vi "zlgcan_demo_USBCANFD_merge.vi"() -> ()   [LabVIEW 2018]
doc: "用于设置CAN通道的初始化参数。\n\n适用的设备：USBCANFD-100U、USBCANFD-200U、USBCANFD-MINI"
uses:
  data_type/ZCAN_InitCAN_setting_USBCANFD.ctl
  data_type/ZCAN_TransmitFD_frame.ctl
  data_type/ZCANDataObj.ctl
panel:
  out "CAN报文显示":string[][](table)
  in  "ZCANDataObj":T1[](array[typedef])
  in  "canfdframe":T2
  out "source":string
  in  "开启CAN":bool
  in  "stop":bool
  in  "?":enum32{"DEMO说明", "设备、通道选择", "参数设置", "状态", "发送"}(tab)
  in  "CAN 通道":u32(ring) items=["0", "1"]
  in  "CAN卡型号":u32(ring)=42 items=["USBCANFD-800U"=59, "USBCANFD-200U"=41, "USBCANFD-100U"=42, "USBCANFD-MINI"=43]
  in  "索引":u32(ring) items=["0", "1", "2", "3", "4", "5", "6", "7", "8"]
  in  "仲裁域波特率":u32(ring)=500000 items=["1Mbps"=1000000, "800kbps"=800000, "500kbps"=500000, "250kbps"=250000, "125kbps"=125000, "100kbps"=100000, "50kbps"=50000]
  in  "数据域波特率":u32(ring)=500000 items=["5Mbps"=5000000, "4Mbps"=4000000, "2Mbps"=2000000, "1Mbps"=1000000, "800kbps"=800000, "500kbps"=500000, "250kbps"=250000, "125kbps"=125000, "100kbps"=100000]
  in  "自定义波特率字符输入":string
  in  "自定义波特率开关":bool
  in  "工作模式":u8(ring) items=["正常", "只听"]
  in  "是否使用电阻":u8(ring)=1 items=["不使用终端电阻", "使用终端电阻"]
  out "error out":errorcluster caption="错误输出"
  out "can_index_handle(out)":u32
  out "Device_handle(out)":u32
  in  "帧类型":u32(ring) items=["标准帧", "扩展帧"]
  in  "帧格式":u32(ring) items=["数据帧", "远程帧"]
  in  "ID":u32=18 format="0x%08x"
  in  "协议":u32(ring) items=["CAN", "CANFD"]
  in  "数据输入":string="11 22 33 44 55 66 77 88"
  in  "CANFD加速？":u32(ring) items=["不加速", "加速"]
  in  "发送":bool
  in  "数据长度":u32(ring)=8 items=["1"=1, "2"=2, "3"=3, "4"=4, "5"=5, "6"=6, "7"=7, "8"=8, "12"=12, "16"=16, "20"=20, "24"=24, "32"=32, "48"=48, "64"=64]
  in  "ZCAN_InitCAN_Setting_USBCANFD":T3
  # "适用的设备：USBCANFD-100U、USBCANFD-200U、USBCANFD-MINI、USBCANFD-800U"
  # "停止程序前，\n请先关闭CAN卡"
  # "1. 确保电脑有VC++ 2005/2008/2010/2013运行库（对应32，64位）,微软常用运行库合集，点击下载（35M）。\n    http://manual.zlg.cn/Public/Uploads/2020-06-05/5ed995c271414.zip"
  # "2，如果打开设备失败，可能原因：\n（1）已经打开过一次，没有正常关闭的情况下，继续点击“打开设备”，是无法打开的。\n     需要USB重新拔插，LABVIEW重启（全部关闭），然后再“打开设备”。\n (2) 项目路径不能有中文繁体。"
  # "使用CAN时，\n两个波特率设置相同即可"
  # "使用ZCANPro软件波特率计算工具计算"
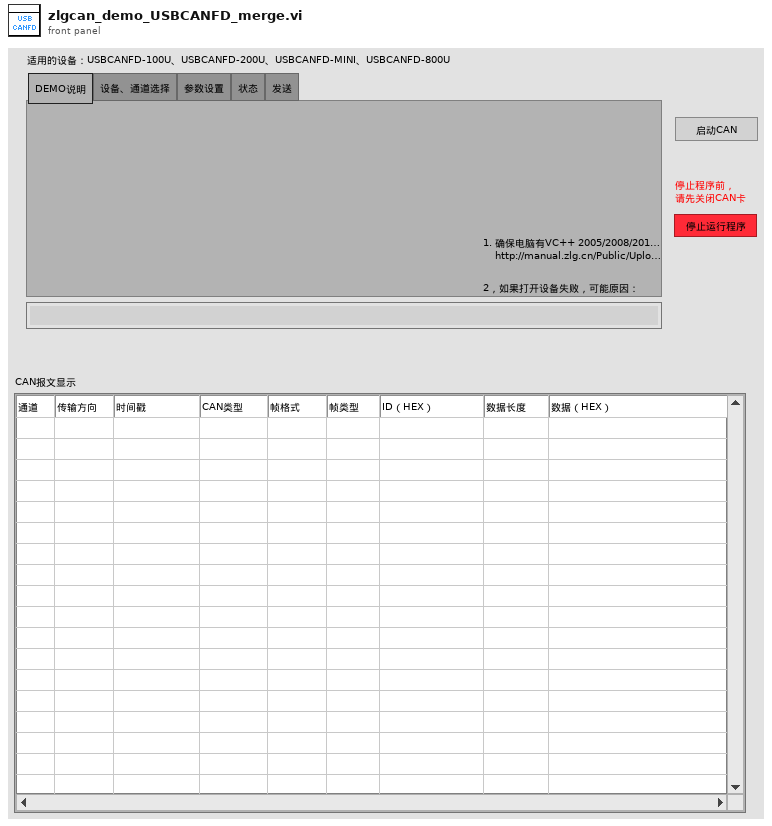
[diagram p1: front panel]
types:
  T1 = typedef "ZCANDataObj.ctl" = cluster{"数据类型":u8, "CAN通道号":u8, "rawVal(未使用)":u16, "extraData[4]（未使用）":cluster{"[0]":u8, "[1]":u8, "[2]":u8, "[3]":u8}, "canCANFDData":cluster{"时间戳+混合标志位":cluster{"时间戳":u64, "混合标志位":u32}, "extraData[4]（未使用）":cluster{"[0]":u8, "[1]":u8, "[2]":u8, "[3]":u8}, "frame":cluster{"can_id":u32, "数据长度":u8, "CANFD加速？":u8, "__res0":u8, "__res1":u8, "data":cluster{"CAN数据[0]":u8, "CAN数据[1]":u8, "CAN数据[2]":u8, "CAN数据[3]":u8, "CAN数据[4]":u8, "CAN数据[5]":u8, "CAN数据[6]":u8, "CAN数据[7]":u8, "CAN数据[8]":u8, "CAN数据[9]":u8, "CAN数据[10]":u8, "CAN数据[11] ":u8, "CAN数据[12] ":u8, "CAN数据[13] ":u8, "CAN数据[14] ":u8, "CAN数据[15] ":u8, "CAN数据[16]":u8, "CAN数据[17]":u8, "CAN数据[18]":u8, "CAN数据[19]":u8, "CAN数据[20]":u8, "CAN数据[21]":u8, "CAN数据[22]":u8, "CAN数据[23]":u8, "CAN数据[24] ":u8, "CAN数据[25]":u8, "CAN数据[26]":u8, "CAN数据[27]":u8, "CAN数据[28]":u8, "CAN数据[29]":u8, "CAN数据[30]":u8, "CAN数据[31]":u8, "CAN数据[32]":u8, "CAN数据[33]":u8, "CAN数据[34]":u8, "CAN数据[35]":u8, "CAN数据[36]":u8, "CAN数据[37]":u8, "CAN数据[38]":u8, "CAN数据[39]":u8, "CAN数据[40]":u8, "CAN数据[41]":u8, "CAN数据[42]":u8, "CAN数据[43]":u8, "CAN数据[44]":u8, "CAN数据[45]":u8, "CAN数据[46]":u8, "CAN数据[47]":u8, "CAN数据[48]":u8, "CAN数据[49]":u8, "CAN数据[50]":u8, "CAN数据[51]":u8, "CAN数据[52]":u8, "CAN数据[53]":u8, "CAN数据[54]":u8, "CAN数据[55]":u8, "CAN数据[56]":u8, "CAN数据[57]":u8, "CAN数据[58]":u8, "CAN数据[59]":u8, "CAN数据[60]":u8, "CAN数据[61]":u8, "CAN数据[62]":u8, "CAN数据[63]":u8}}}, "Reserve":u32}
  T2 = typedef "ZCAN_TransmitFD_frame.ctl" = cluster{"帧类型":u32, "帧格式":u32, "ID":u32, "数据长度":u8, "CANFD加速？":u8, "DATA":cluster{"CAN数据[0]":u8, "CAN数据[1]":u8, "CAN数据[2]":u8, "CAN数据[3]":u8, "CAN数据[4]":u8, "CAN数据[5]":u8, "CAN数据[6]":u8, "CAN数据[7]":u8, "CAN数据[8]":u8, "CAN数据[9]":u8, "CAN数据[10]":u8, "CAN数据[11] ":u8, "CAN数据[12] ":u8, "CAN数据[13] ":u8, "CAN数据[14] ":u8, "CAN数据[15] ":u8, "CAN数据[16]":u8, "CAN数据[17]":u8, "CAN数据[18]":u8, "CAN数据[19]":u8, "CAN数据[20]":u8, "CAN数据[21]":u8, "CAN数据[22]":u8, "CAN数据[23]":u8, "CAN数据[24] ":u8, "CAN数据[25]":u8, "CAN数据[26]":u8, "CAN数据[27]":u8, "CAN数据[28]":u8, "CAN数据[29]":u8, "CAN数据[30]":u8, "CAN数据[31]":u8, "CAN数据[32]":u8, "CAN数据[33]":u8, "CAN数据[34]":u8, "CAN数据[35]":u8, "CAN数据[36]":u8, "CAN数据[37]":u8, "CAN数据[38]":u8, "CAN数据[39]":u8, "CAN数据[40]":u8, "CAN数据[41]":u8, "CAN数据[42]":u8, "CAN数据[43]":u8, "CAN数据[44]":u8, "CAN数据[45]":u8, "CAN数据[46]":u8, "CAN数据[47]":u8, "CAN数据[48]":u8, "CAN数据[49]":u8, "CAN数据[50]":u8, "CAN数据[51]":u8, "CAN数据[52]":u8, "CAN数据[53]":u8, "CAN数据[54]":u8, "CAN数据[55]":u8, "CAN数据[56]":u8, "CAN数据[57]":u8, "CAN数据[58]":u8, "CAN数据[59]":u8, "CAN数据[60]":u8, "CAN数据[61]":u8, "CAN数据[62]":u8, "CAN数据[63]":u8}}
  T3 = typedef "ZCAN_InitCAN_setting_USBCANFD.ctl" = cluster{"abitbaud":u32, "dbitbaud":u32, "baud_rate_custom？":bool, "RateCustom":string, "mode":u8}
  T4 = cluster{"[0]":u32, "[1]":u32, "[2]":u32, "[3]":u32, "[4]":u32, "[5]":u32, "[6]":u32, "[7]":u32, "[8]":u32, "[9]":u32, "[10]":u32, "[11]":u32, "[12]":u32, "[13]":u32, "[14]":u32, "[15]":u32, "[16]":u32, "[17]":u32, "[18]":u32, "[19]":u32, "[20]":u32, "[21]":u32, "[22]":u32, "[23]":u32, "[24]":u32, "[25]":u32, "[26]":u32, "[27]":u32, "[28]":u32, "[29]":u32, "[30]":u32, "[31]":u32, "[32]":u32, "[33]":u32, "[34]":u32, "[35]":u32, "[36]":u32, "[37]":u32, "[38]":u32, "[39]":u32, "[40]":u32, "[41]":u32, "[42]":u32, "[43]":u32, "[44]":u32, "[45]":u32, "[46]":u32, "[47]":u32, "[48]":u32, "[49]":u32, "[50]":u32, "[51]":u32, "[52]":u32, "[53]":u32, "[54]":u32, "[55]":u32, "[56]":u32, "[57]":u32, "[58]":u32, "[59]":u32, "[60]":u32, "[61]":u32, "[62]":u32, "[63]":u32}
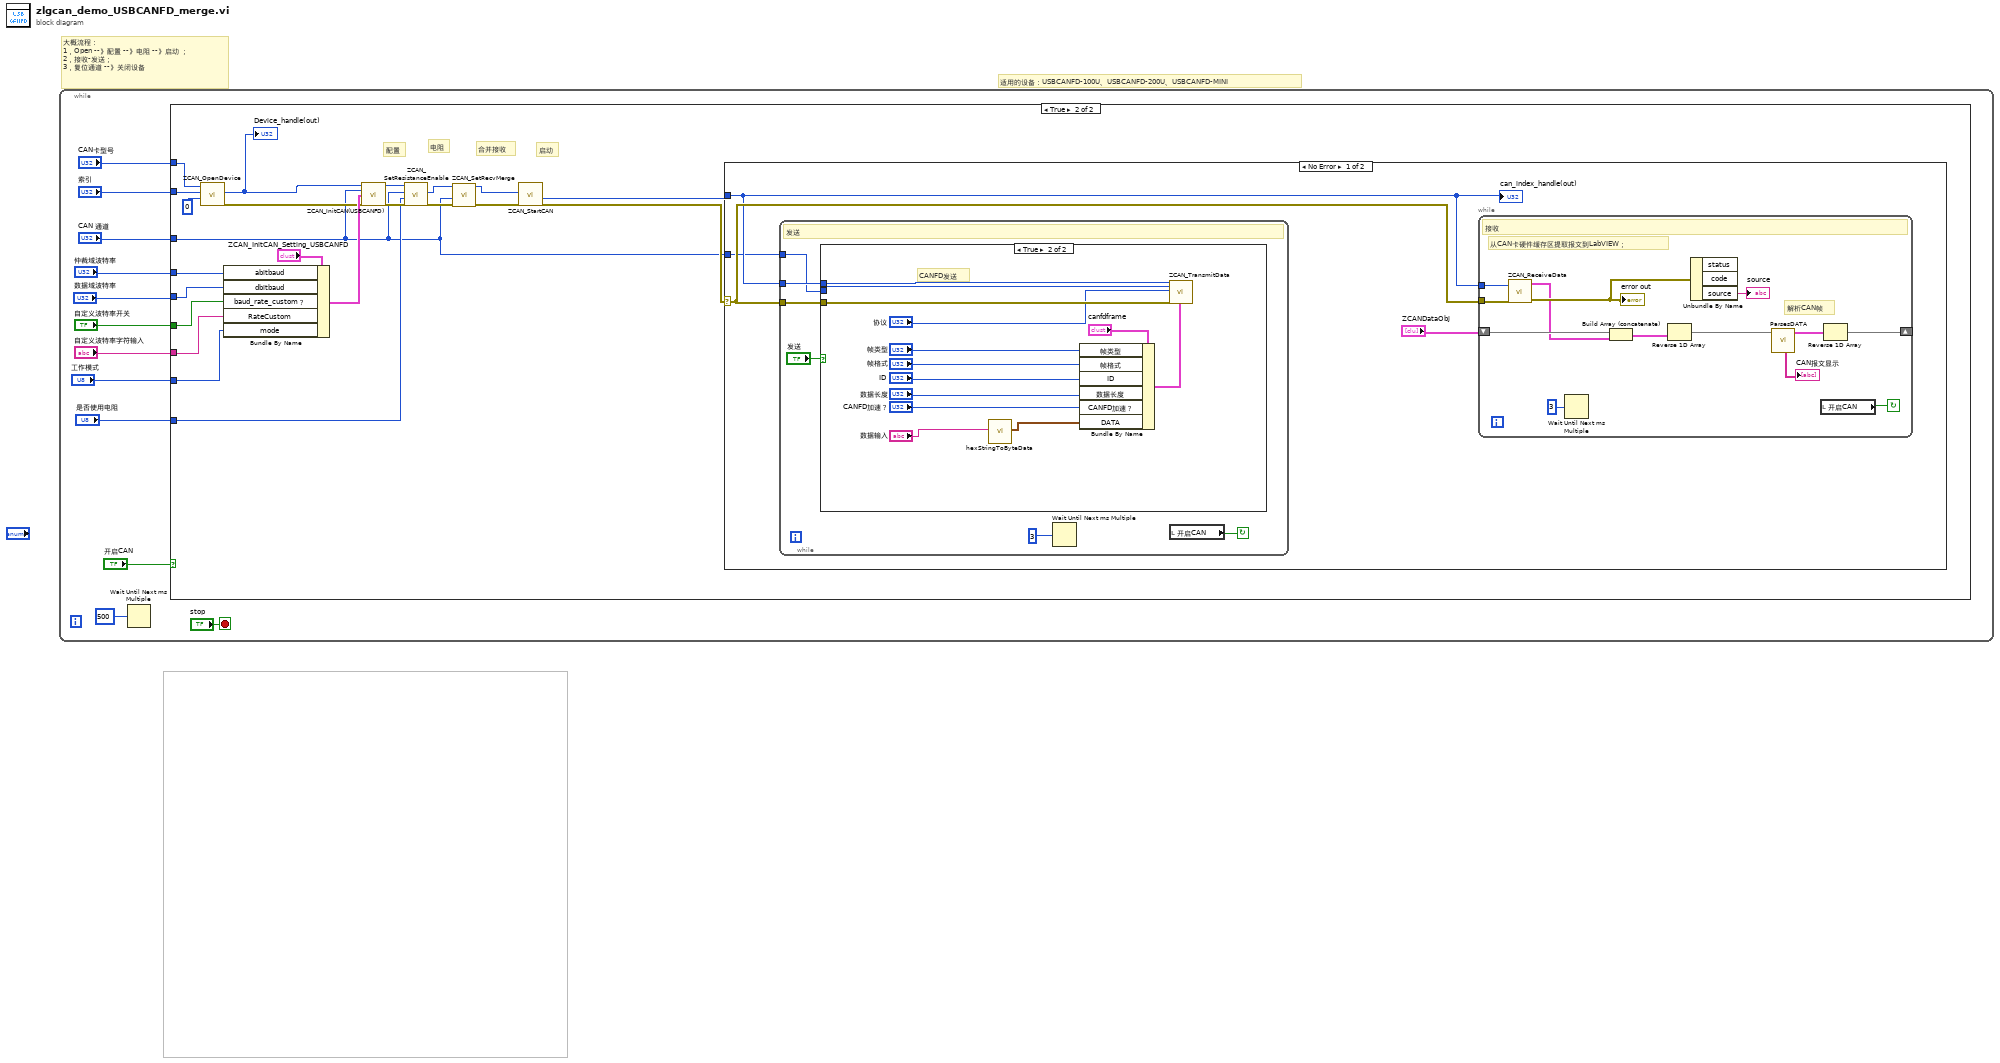
[diagram p0: block diagram]
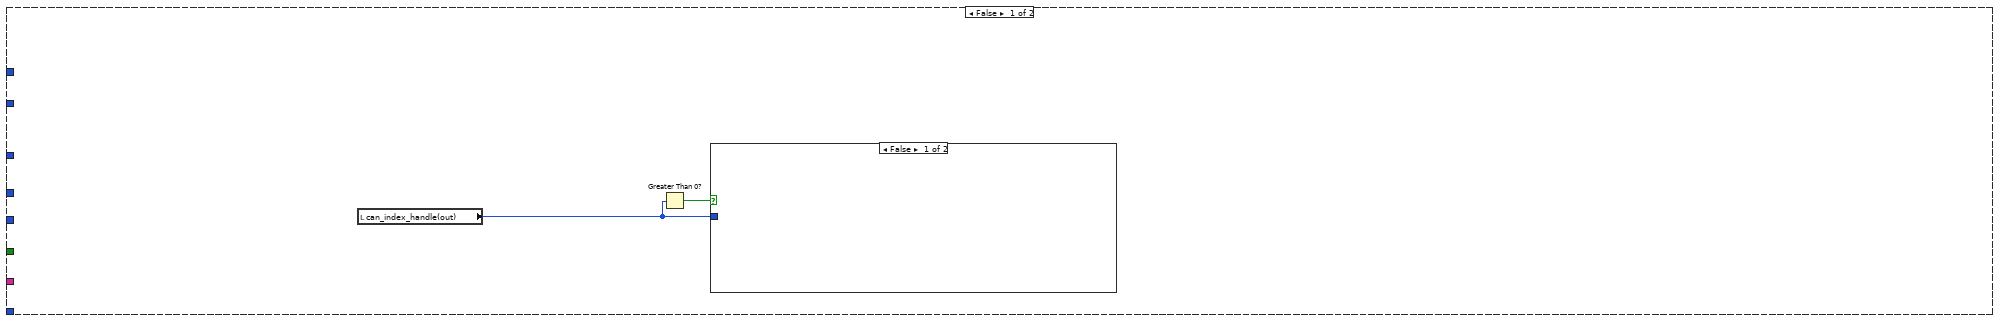
[diagram p2: hidden frame]
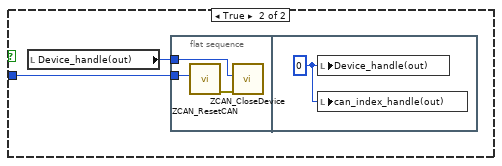
[diagram p3: hidden frame]
diagram:
  # "大概流程：\n1，Open --》配置 --》电阻 --》启动 ；\n2，接收-发送；\n3，复位通道 --》关闭设备"
  # "适用的设备：USBCANFD-100U、USBCANFD-200U、USBCANFD-MINI"
  n1 = while {
    stop <- "stop" stop-if-true
    n2 = Wait Until Next ms Multiple(millisecond multiple=u32 500) -> ()  [unwired: 1 out]
    n3 = case shown="True" "开启CAN" {
      tunnel: "CAN 通道" -> [_ w21]
      tunnel: "仲裁域波特率" -> [_ w35]
      tunnel: "自定义波特率开关" -> [_ w37]
      tunnel: "自定义波特率字符输入" -> [_ w34]
      tunnel: "工作模式" -> [_ w33]
      tunnel: "CAN卡型号" -> [_ w40]
      tunnel: "索引" -> [_ w41]
      tunnel: "数据域波特率" -> [_ w36]
      tunnel: "是否使用电阻" -> [_ w30]
      frame False {
        # "关闭CAN卡"
        n4 = local read "can_index_handle(out)"() -> (w13:u32)
        n5 = Greater Than 0?(x=w13) -> (x > 0?=w14:bool)
        n6 = case shown="False" w14 {
          tunnel: w13 -> [_ w16]
          frame False {
          }
          frame True {
            n7 = local read "Device_handle(out)"() -> (w15:u32)
            n8 = flat-sequence {
              tunnel: w16 -> [w18]
              tunnel: w15 -> [w17]
              frame #0 {
                n9 = call "ZCAN_ResetCAN.vi"("can_handle"=w18) -> ("error out"=w19:errorcluster)  [unwired: 9 in, 1 out]
                n10 = call "ZCAN_CloseDevice.vi"("error in (no error)"=w19, "device_handle"=w17) -> ()  [unwired: 8 in, 2 out]
              }
              frame #1 {
                w20 = u32 0 ("can_index_handle(out)")
                n11 = local write "Device_handle(out)"(w20) -> ()
                n12 = local write "can_index_handle(out)"(w20) -> ()
              }
            }
          }
        }
      }
      frame True {
        # "合并接收"
        # "启动"
        # "电阻"
        # "配置"
        n13 = call "ZCAN_OpenDevice.vi"("reserved"=0, "device_index"=w41, "device_type"=w40) -> ("error out"=w29:errorcluster, "DEVICE_HANDLE"=w28:u32)  [unwired: 7 in]
        "Device_handle(out)" <- w28
        n14 = Bundle By Name(cluster="ZCAN_InitCAN_Setting_USBCANFD", "abitbaud"=w35, "dbitbaud"=w36, "baud_rate_custom？"=w37, "RateCustom"=w34, "mode"=w33) -> (w32:T3)
        n15 = call "ZCAN_InitCAN(USBCANFD).vi"("device_hande"=w28, "can_index"=w21, "ZCAN_InitCAN_Setting_USBCANFD"=w32, "error in (no error)"=w29) -> ("can_index_handle"=w26:u32, "error out"=w31:errorcluster)  [unwired: 10 in]
        n16 = call "ZCAN_SetResistanceEnable.vi"("error in (no error)"=w31, "enable"=w30, "can_index"=w21, "can_index_handle"=w26) -> ("error out"=w22:errorcluster, "can_index_handle(out)"=w25:u32)  [unwired: 6 in]
        n17 = call "ZCAN_SetRecvMerge.vi"("device_handle"=w25, "can通道"=w21, "error in (no error)"=w22) -> ("device_handle(out)"=w24:u32, "error out"=w23:errorcluster)  [unwired: 5 in, 1 out]
        n18 = call "ZCAN_StartCAN.vi"("error in (no error)"=w23, "can_index_handle"=w24) -> ("error out"=w27:errorcluster, "can_index_handle(out)"=w39:u32)  [unwired: 7 in, 1 out]
        n19 = case shown="No Error" w27 {
          selector: w27 -> [w46 _]
          tunnel: w39 -> [w45 _]
          tunnel: w21 -> [w43 _]
          frame No Error {
            n20 = while {
              tunnel: w45 -> [w63]
              tunnel: w46 -> [w61]
              tunnel: w43 -> [w60]
              stop <- w62 continue-if-true
              # "发送"
              n21 = case shown="True" "发送" {
                tunnel: w63 -> [_ w74]
                tunnel: w61 -> [_ w75]
                tunnel: w60 -> [_ w68]
                frame False {
                }
                frame True {
                  # "CANFD发送"
                  n22 = call "hexStringToByteData.vi"("数据输入 2"="数据输入") -> ("CANFD_data"=w66:T4)  [unwired: 9 in, 1 out]
                  n23 = Bundle By Name(cluster="canfdframe", "帧类型"="帧类型", "帧格式"="帧格式", "ID"="ID", "数据长度"="数据长度", "CANFD加速？"="CANFD加速？", "DATA"=w66) -> (w70:T2)
                  n24 = call "ZCAN_TransmitData.vi"("can_index_handle"=w74, "CAN通道号"=w68, "帧类型"="协议", "error in (no error)"=w75, "canfd_frame"=w70) -> ()  [unwired: 14 in, 1 out]
                }
              }
              n25 = Wait Until Next ms Multiple(millisecond multiple=u32 3) -> ()  [unwired: 1 out]
              n26 = local read "开启CAN"() -> (w62:bool)
            }
            n27 = while {
              tunnel: w46 -> [w58]
              tunnel: w45 -> [w57]
              shift-right: [w49] -> _
              shift-left: "ZCANDataObj" -> [w55]
              stop <- w56 continue-if-true
              # "从CAN卡硬件缓存区提取报文到LabVIEW；"
              # "解析CAN帧"
              # "接收"
              n28 = call "ZCAN_ReceiveData.vi"("error in (no error)"=w58, "can_handle"=w57) -> ("error out"=w52:errorcluster, "ZCANDataObj（out）"=w51:T1[])  [unwired: 2 in, 1 out]
              "error out" <- w52
              n29 = Wait Until Next ms Multiple(millisecond multiple=u32 3) -> ()  [unwired: 1 out]
              n30 = Build Array (concatenate)(w55, w51) -> (w54:T1[])
              n31 = Reverse 1D Array(array=w54) -> (reversed array=w50:T1[])
              n32 = Unbundle By Name(w52) -> ("source"=→"source":string)  [unwired: 2 out]
              n33 = call "ParsesDATA.vi"("ZCANDataObj"=w50) -> ("ZCANDataObj(out)"=w48:T1[], "CAN报文显示"=→"CAN报文显示":string[][])  [unwired: 9 in]
              n34 = local read "开启CAN"() -> (w56:bool)
              n35 = Reverse 1D Array(array=w48) -> (reversed array=w49:T1[])
            }
            "can_index_handle(out)" <- w45
          }
          frame Error {
          }
        }
      }
    }
  }
